vi "General LS Linear Fit (obs).vi"(0 "H":dbl[][](array[numeric]) format="%0.2f", 1 "Y":dbl[](array[numeric]) format="%0.2f", 2 "covariance selector":T1(ring), 3 "algorithm":T3(ring), 4 "Standard Deviation":dbl[](array[numeric]) format="%0.2f") -> (5 "Covariance":T2, 6 "Coefficients":dbl[](array[numeric]) format="%0.2f", 7 "Best Fit":dbl[](array[numeric]) format="%0.2f", 8 "mse":dbl format="%0.2f", 9 "error":i32)   [LabVIEW 2017, in "NI_AALPro.lvlib"]
doc: "Finds the k-dimension linear curve values and the set of k-dimension linear fit coefficients, which describe the k-dimension linear curve that best represents the input data set using the least-squares solution."
uses:
  NI_AALPro.lvlib
  RealMatrix.ctl
  lvanlys.dll
  NI_Matrix.lvlib
panel:
  # "General LS Linear Fit (obsolete)"
  # "This VI is obsolete !!!\nYou should replace this VI in your diagram with the General LS Linear Fit VI.  \n\nNOTE: If you have wired to the Standard Deviation input of this obsolete VI, \n           please be aware that the new General LS Linear Fit VI accepts a Weight \n           input instead of Standard Deviation.  The equation that you can use to \n           map Standard Deviation to Weight is:\n\n             \t\tWeight = 1 / (Standard Deviation)^2"
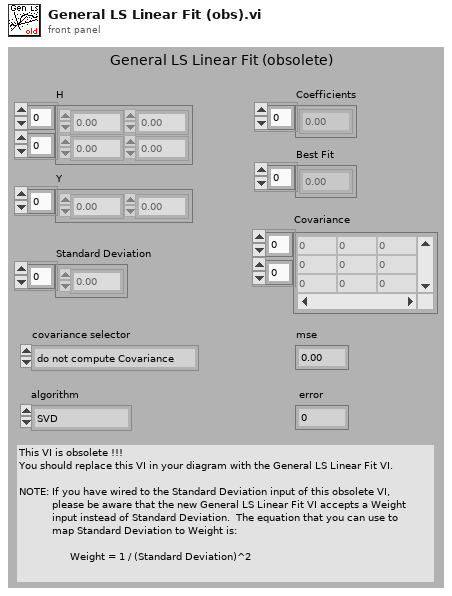
[diagram p1: front panel]
types:
  T1 = enum32{"do not compute Covariance", " compute Covariance"}
  T2 = typedef "NI_Matrix.lvlib/RealMatrix.ctl" = dbl[][]
  T3 = enum32{"SVD", "Givens", "Givens2", "Householder", "LU Decomposition", "Cholesky"}
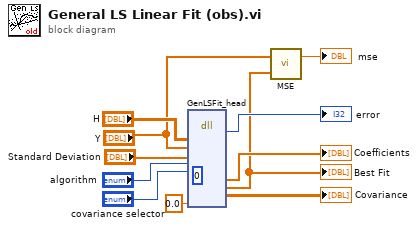
[diagram p0: block diagram]
diagram:
  (unwired) 0
  n1 = dll-call lib="C:/Program Files/National Instruments/LabVIEW 2017/resource/lvanlys.*" fn="GenLSFit_head"("H"="H", "Y Values"="Y", "Standard Deviation"="Standard Deviation", "algorithm"="algorithm", "covariance selector"="covariance selector", "mse"=0.0) -> (→"error":i32, "CoefH"=→"Coefficients":dbl[], "BestFitH"=w3:dbl[], "CovarH"=→"Covariance":dbl[][])  [unwired: 12 in, 2 out]
  "Best Fit" <- w3
  n2 = call "MSE.vi"("X Values"=w3, "Y Values"="Y") -> ("mse"=→"mse":dbl)  [unwired: 1 out]
